vi "Update Card with De and Activate.vi"(7 "BME_DG_System in":refnum<class "BME_DG_System.lvclass">, 8 "error in (no error)":errorcluster, 10 "ResetCounter":enum16{"Slaves only", "Slaves & Master"}(ring)=enum."Slaves & Master", 11 "BME_DG_Chnl in":refnum<class "BME_DG_Chnl.lvclass">) -> (0 "error out":errorcluster, 5 "BME_DG_System out":refnum<class "BME_DG_System.lvclass">)   [LabVIEW 2009, in "BME_DG_Chnl.lvclass"]
doc: "The VI modifies delay settings of a channel.\nAt first step if master card is activated this VI deactivates it, also its own card.\nThen it modifies channel delay settings. After this activate the previosly active cards again. \n\nAutor: Alexander Kessler\nalexander.kessler@uni-jena.de\n\nGNU license.\nHelmholtz-Institut-Jena"
uses:
  BME_DG_Chnl.lvclass
  BME_DG_System/BME_DG_System.lvclass
  BME_DG_Chnl.lvclass/BME_DG_Chnl.ctl
  BME_DG_Base/BME_DG_Base.lvclass
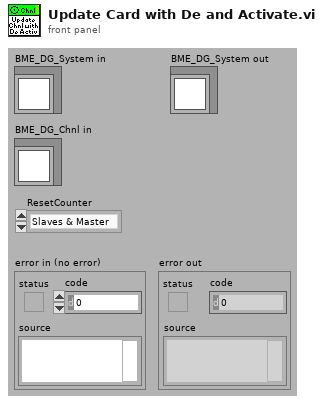
[diagram p1: front panel]
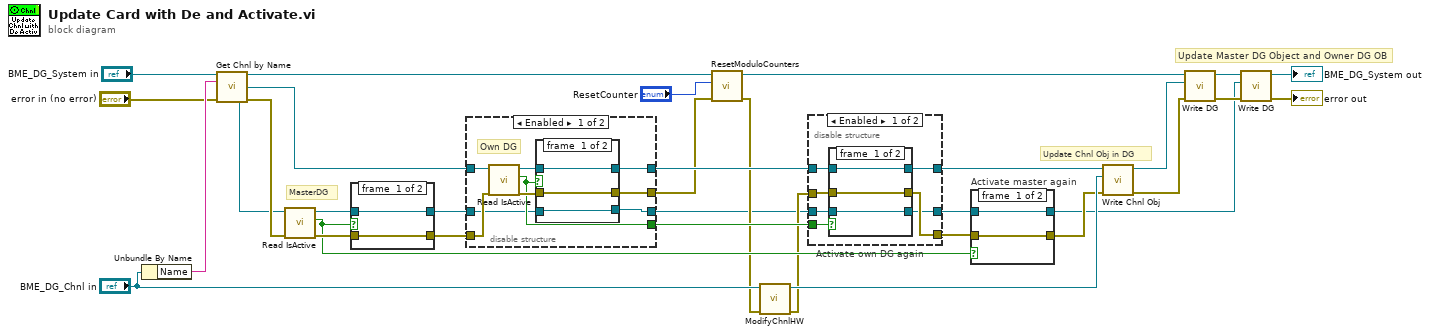
[diagram p0: block diagram]
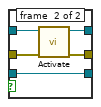
[diagram p2: hidden frame]
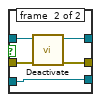
[diagram p4: hidden frame]
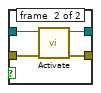
[diagram p6: hidden frame]
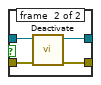
[diagram p7: hidden frame]
diagram:
  # "MasterDG"
  # "Update Chnl Obj in DG"
  # "Update Master DG Object and Owner DG OB"
  n1 = Unbundle By Name("BME_DG_Chnl in") -> ("Name"=w13:string)
  n2 = call "Get Chnl by Name.vi"("BME_DG_System in"="BME_DG_System in", "Chnl Name"=w13, "error in (no error)"="error in (no error)") -> ("BME_DG_System out"=w7:refnum<class "BME_DG_System.lvclass">, "Owner DG"=w10:refnum<class "BME_DG_Base.lvclass">, "Master DG"=w9:refnum<class "BME_DG_Base.lvclass">, "error out"=w11:errorcluster)  [unwired: 7 in, 2 out]
  n3 = call-dynamic "Read IsActive.vi"("error in (no error)"=w11, "BME_DG_Base in"=w9) -> ("error out"=w28:errorcluster, "Active?"=w27:bool, "BME_DG_Base out"=w29:refnum<class "BME_DG_Base.lvclass">)  [unwired: 7 in]
  n4 = case shown="True" w27 {
    tunnel: w29 -> [w34 w39]
    tunnel: w28 -> [w35 w38]
    tunnel: [w35 w37] -> w24
    tunnel: [w34 w36] -> w3
    frame #0 {
    }
    frame #1 {
      n5 = call-dynamic "Deactivate.vi"("error in (no error)"=w38, "BME_DG_Base in"=w39) -> ("error out"=w37:errorcluster, "BME_DG_Base out"=w36:refnum<class "BME_DG_Base.lvclass">)  [unwired: 8 in]
    }
  }
  n6 = disable-structure shown="Enabled" {
    disable-tunnel: [w46 w58] -> w26
    disable-tunnel: [w45 _] -> w25
    disable-tunnel: w24 -> [w44 w59]
    disable-tunnel: [w43 w59] -> w8
    disable-tunnel: w10 -> [w42 w58]
    disable-tunnel: w3 -> [w41 w57]
    disable-tunnel: [w40 w57] -> w1
    frame #0 {
      # "Own DG"
      n7 = call-dynamic "Read IsActive.vi"("error in (no error)"=w44, "BME_DG_Base in"=w42) -> ("error out"=w47:errorcluster, "Active?"=w45:bool, "BME_DG_Base out"=w48:refnum<class "BME_DG_Base.lvclass">)  [unwired: 7 in]
      n8 = case shown="True" w45 {
        tunnel: w48 -> [w51 w56]
        tunnel: w47 -> [w50 w55]
        tunnel: [w51 w54] -> w46
        tunnel: [w50 w53] -> w43
        tunnel: w41 -> [w49 w52]
        tunnel: [w49 w52] -> w40
        frame #0 {
        }
        frame #1 {
          n9 = call-dynamic "Deactivate.vi"("error in (no error)"=w55, "BME_DG_Base in"=w56) -> ("error out"=w53:errorcluster, "BME_DG_Base out"=w54:refnum<class "BME_DG_Base.lvclass">)  [unwired: 8 in]
        }
      }
    }
    frame #1 {
    }
  }
  n10 = call "ResetModuloCounters.vi"("error in (no error)"=w8, "Enum"="ResetCounter", "BME_DG_System in"=w7) -> ("error out"=w4:errorcluster, "BME_DG_System out"=w6:refnum<class "BME_DG_System.lvclass">)  [unwired: 7 in]
  n11 = call-dynamic "ModifyChnlHW.vi"("error in (no error)"=w4, "BME_DG_Chnl in"="BME_DG_Chnl in") -> ("error out"=w23:errorcluster, "BME_DG_Chnl out"=w32:refnum<class "BME_DG_Chnl.lvclass">)  [unwired: 8 in]
  n12 = disable-structure shown="Enabled" {
    disable-tunnel: w26 -> [w66 w76]
    disable-tunnel: w25 -> [w65 _]
    disable-tunnel: w23 -> [w62 w77]
    disable-tunnel: [w64 w77] -> w22
    disable-tunnel: [w63 w76] -> w16
    disable-tunnel: [w60 w75] -> w2
    disable-tunnel: w1 -> [w61 w75]
    frame #0 {
      n13 = case "Activate own DG again" shown="True" w65 {
        tunnel: w66 -> [w68 w74]
        tunnel: w62 -> [w69 w73]
        tunnel: [w69 w71] -> w64
        tunnel: [w68 w72] -> w63
        tunnel: w61 -> [w67 w70]
        tunnel: [w67 w70] -> w60
        frame #0 {
        }
        frame #1 {
          n14 = call-dynamic "Activate.vi"("error in (no error)"=w73, "BME_DG_Base in"=w74) -> ("error out"=w71:errorcluster, "BME_DG_Base out"=w72:refnum<class "BME_DG_Base.lvclass">)  [unwired: 8 in]
        }
      }
    }
    frame #1 {
    }
  }
  n15 = case "Activate master again" shown="True" w27 {
    tunnel: w2 -> [w79 w83]
    tunnel: [w78 w81] -> w21
    tunnel: [w79 w82] -> w17
    tunnel: w22 -> [w78 w80]
    frame #0 {
    }
    frame #1 {
      n16 = call-dynamic "Activate.vi"("error in (no error)"=w80, "BME_DG_Base in"=w83) -> ("error out"=w81:errorcluster, "BME_DG_Base out"=w82:refnum<class "BME_DG_Base.lvclass">)  [unwired: 8 in]
    }
  }
  n17 = call-dynamic "Write Chnl Obj.vi"("error in (no error)"=w21, "BME_DG_Chnl"=w32, "BME_DG_Base in"=w16) -> ("error out"=w19:errorcluster, "BME_DG_Base out"=w15:refnum<class "BME_DG_Base.lvclass">)  [unwired: 7 in]
  n18 = call "Write DG.vi"("error in (no error)"=w19, "BME_DG_Base"=w15, "BME_DG_System in"=w6) -> ("error out"=w18:errorcluster, "BME_DG_System out"=w20:refnum<class "BME_DG_System.lvclass">)  [unwired: 7 in]
  n19 = call "Write DG.vi"("error in (no error)"=w18, "BME_DG_Base"=w17, "BME_DG_System in"=w20) -> ("error out"=→"error out":errorcluster, "BME_DG_System out"=→"BME_DG_System out":refnum<class "BME_DG_System.lvclass">)  [unwired: 7 in]
